vi "ReverseQuestionMark.vi"(8 "notor speed":dbl, 10 "wanted in":dbl, 11 "refnum name in":string="My Motor RefNum") -> (0 "notor speed 2":dbl, 2 "wanted out":dbl, 3 "refnum name out":string="My Motor RefNum")   [LabVIEW 2020]
uses:
  <vilib>/Rock Robotics/WPI/ThirdParty/Phoenix-LabVIEW/Motor Controller/Get/CTRE_Phoenix_MotorController_GetSelectedSensorData.vi
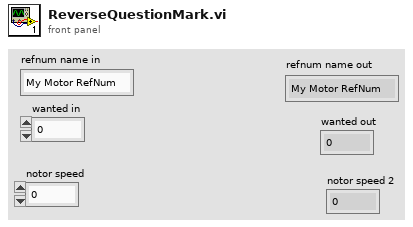
[diagram p1: front panel]
types:
  T1 = typedef "WPI_MotorControlDeviceRef.ctl" = cluster{"DeviceStatus":errorcluster, "Type":T2, "PWM":cluster{"PWM Channel":T3, "DeadBand":T4}, "CAN":cluster{"Device Number":u8, "SetOutput VI Ref":variant, "GetOutput VI Ref":variant, "Enable VI Ref":variant, "Disable VI Ref":variant, "Data":variant}, "Invert":bool, "DIO PWM":cluster{"PWM \"Enable\" Channel":T3, "DIOChannel":T5, "PWM Rate":dbl}}
  T2 = typedef "WPI_MotorControlType.ctl" = enum16{"PWM", "CAN", "DIO PWM"}
  T3 = typedef "FPGA_DIOPWMChannel.ctl" = enum8{"PWM 0", "PWM 1", "PWM 2", "PWM 3", "PWM 4", "PWM 5", "PWM 6", "PWM 7", "PWM 8", "PWM 9", "PWM MXP 0", "PWM MXP 1", "PWM MXP 2", "PWM MXP 3", "PWM MXP 4", "PWM MXP 5", "PWM MXP 6", "PWM MXP 7", "PWM MXP 8", "PWM MXP 9", "Invalid"}
  T4 = typedef "WPI_PWMDeadband.ctl" = cluster{"Name":string, "maxPositivePwm":i32, "minPositivePwm":i32, "centerPwm":i32, "maxNegativePwm":i32, "minNegativePwm":i32, "angularRange":u16}
  T5 = typedef "FPGA_DIOChannel.ctl" = enum8{"DIO 0", "DIO 1", "DIO 2", "DIO 3", "DIO 4", "DIO 5", "DIO 6", "DIO 7", "DIO 8", "DIO 9", "DIO MXP 0", "DIO MXP 1", "DIO MXP 2", "DIO MXP 3", "DIO MXP 4", "DIO MXP 5", "DIO MXP 6", "DIO MXP 7", "DIO MXP 8", "DIO MXP 9", "DIO MXP 10", "DIO MXP 11", "DIO MXP 12", "DIO MXP 13", "DIO MXP 14", "DIO MXP 15", "SPI Port CS1", "SPI Port CS2", "SPI Port CS3", "SPI Port MISO", "SPI Port MOSI", "Invalid"}
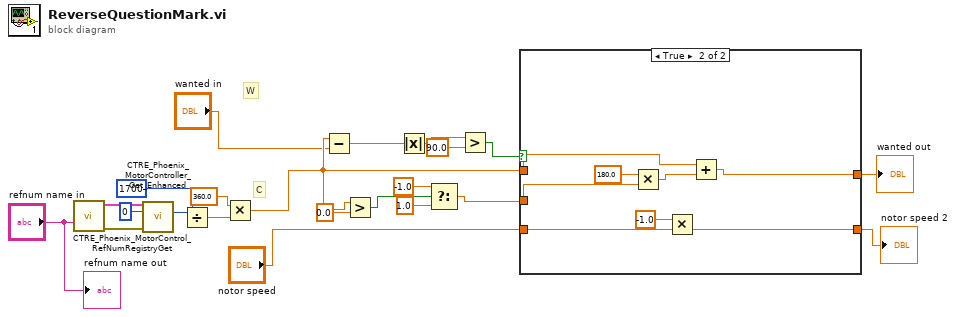
[diagram p0: block diagram]
diagram:
  # "W"
  # "C"
  n1 = call <vilib>:"CTRE_Phoenix_MotorControl_RefNumRegistryGet.vi"("refnum name"="refnum name in") -> ("error out"=w6:errorcluster, "PhoenixMotorControlDevRef"=w5:T1)  [unwired: 9 in]
  n2 = call-poly <vilib>:"CTRE_Phoenix_MotorController_Get_Enhanced.vi"("PhoenixMotorControlDevRef"=w5, "pidLoopIdx"=u32 0, "error in"=w6) -> ("Position (Raw Sensor Units)"=w7:i32)  [unwired: 9 in, 3 out]
  n3 = Divide(x=w7, y=1700) -> (x/y=w8:dbl)
  n4 = Multiply(x=360.0, y=w8) -> (x*y=w21:dbl)
  n5 = Subtract(x=w21, y="wanted in") -> (x-y=w12:dbl)
  n6 = Greater?(x=w21, y=0.0) -> (0:w16:bool)
  n7 = Absolute Value(x=w12) -> (abs(x)=w13:dbl)
  n8 = Select(t=-1.0, s=w16, f=1.0) -> (s? t:f=w20:dbl)
  n9 = Greater?(x=w13, y=90.0) -> (0:w19:bool)
  n10 = case shown="True" w19 {
    tunnel: w20 -> [_ w32]
    tunnel: w21 -> [w24 w29]
    tunnel: [w24 w28] -> w22
    tunnel: [w23 w26] -> w2
    tunnel: "notor speed" -> [w23 w27]
    frame False {
    }
    frame True {
      n11 = Multiply(x=180.0, y=w32) -> (x*y=w30:dbl)
      n12 = Multiply(x=-1.0, y=w27) -> (x*y=w26:dbl)
      n13 = Add(x=w29, y=w30) -> (x+y=w28:dbl)
    }
  }
  "wanted out" <- w22
  "notor speed 2" <- w2
  "refnum name out" <- "refnum name in"
